vi "Main.vi"() -> ()   [LabVIEW 2012]
uses:
  States Main.ctl
  States SubVi.ctl
panel:
  out "error out":errorcluster
  in  "Exit":bool
  in  "Close":bool
  in  "Stop":bool
  in  "Open":bool
  in  "Start":bool
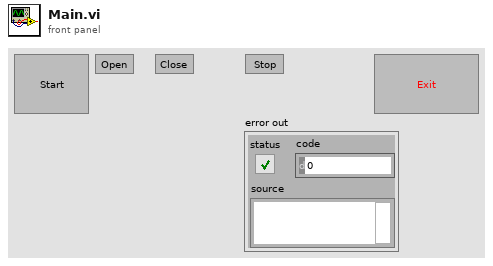
[diagram p1: front panel]
types:
  T1 = typedef "States SubVi.ctl" = enum16{"def", "Random", "Exit"}
  T2 = typedef "States Main.ctl" = enum16{"def", "Start", "Open", "Close", "Stop", "Exit"}
  T3 = enum32{"Invalid", "Standard", "Closed", "Hidden", "Minimized", "Maximized"}
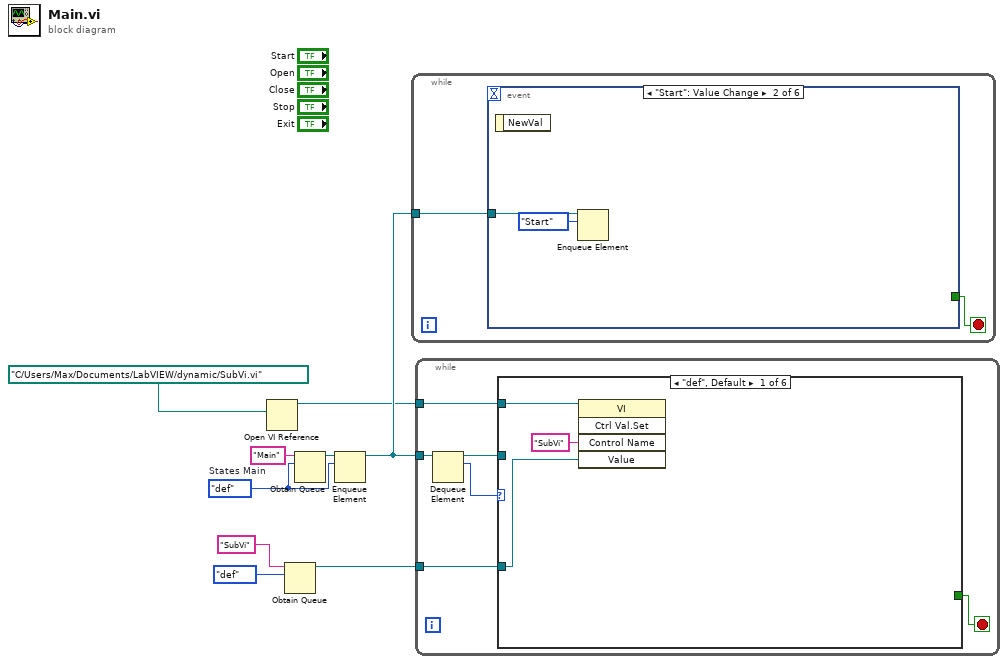
[diagram p0: block diagram]
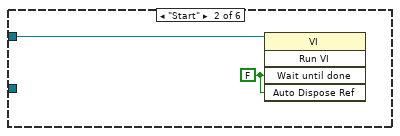
[diagram p2: hidden frame]
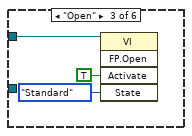
[diagram p3: hidden frame]
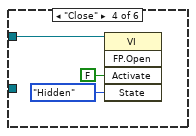
[diagram p4: hidden frame]
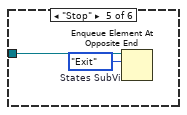
[diagram p5: hidden frame]
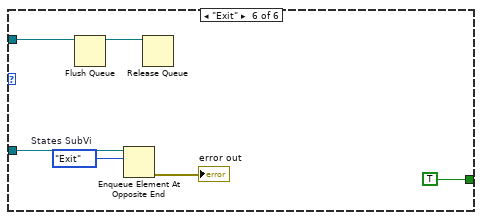
[diagram p6: hidden frame]
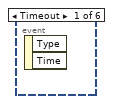
[diagram p7: hidden frame]
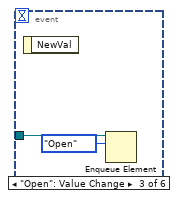
[diagram p8: hidden frame]
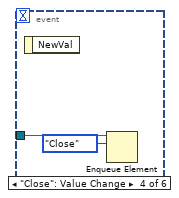
[diagram p9: hidden frame]
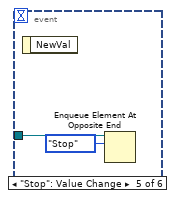
[diagram p10: hidden frame]
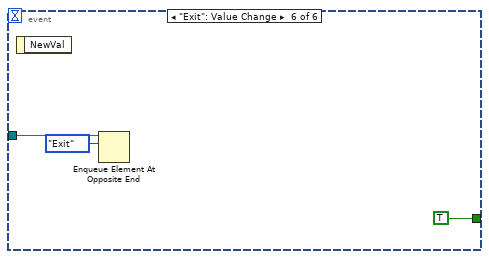
[diagram p11: hidden frame]
diagram:
  w7 = States_Main."def"  # States Main
  n1 = Open VI Reference(vi path=path "C:/Users/Max/Documents/LabVIEW/dynamic/SubVi.vi") -> (vi reference=w4:refnum<vi>)  [unwired: 5 in, 1 out]
  n2 = Obtain Queue(name (unnamed)="SubVi", element data type=States_SubVi."def" ("States SubVi")) -> (queue out=w1:refnum<queue>)  [unwired: 3 in, 2 out]
  n3 = Obtain Queue(name (unnamed)="Main", element data type=w7) -> (queue out=w8:refnum<queue>)  [unwired: 3 in, 2 out]
  n4 = Enqueue Element(queue=w8, element=w7) -> (queue out=w6:refnum<queue>)  [unwired: 2 in, 2 out]
  n5 = while {
    tunnel: w6 -> [w11]
    stop <- w10 stop-if-true
    n6 = event shown="[1] \"Start\": Value Change" {
      selector: _ -> [_ _ _ _ _ _]
      dyn-events: _ -> [_ _ _ _ _ _]
      timeout: _ -> [_ _ _ _ _ _]
      tunnel: w11 -> [_ w13 w15 w17 w19 w22]
      tunnel: [_ _ _ _ _ TRUE] -> w10
      event Timeout {
        n7 = event-data() -> ()  [unwired: 1 in, 2 out]
      }
      event "Start": Value Change {
        n8 = event-data() -> ()  [unwired: 1 in, 1 out]
        n9 = Enqueue Element(queue=w13, element=States_Main."Start") -> ()  [unwired: 2 in, 3 out]
      }
      event "Open": Value Change {
        n10 = event-data() -> ()  [unwired: 1 in, 1 out]
        n11 = Enqueue Element(queue=w15, element=States_Main."Open") -> ()  [unwired: 2 in, 3 out]
      }
      event "Close": Value Change {
        n12 = event-data() -> ()  [unwired: 1 in, 1 out]
        n13 = Enqueue Element(queue=w17, element=States_Main."Close") -> ()  [unwired: 2 in, 3 out]
      }
      event "Stop": Value Change {
        n14 = event-data() -> ()  [unwired: 1 in, 1 out]
        n15 = Enqueue Element At Opposite End(queue=w19, element=States_Main."Stop") -> ()  [unwired: 2 in, 3 out]
      }
      event "Exit": Value Change {
        n16 = event-data() -> ()  [unwired: 1 in, 1 out]
        n17 = Enqueue Element At Opposite End(queue=w22, element=States_Main."Exit") -> ()  [unwired: 2 in, 3 out]
      }
    }
  }
  n18 = while {
    tunnel: w6 -> [w28]
    tunnel: w4 -> [w26]
    tunnel: w1 -> [w23]
    stop <- w24 stop-if-true
    n19 = Dequeue Element(queue=w28) -> (queue out=w25:refnum<queue>, element=w27:T2)  [unwired: 2 in, 2 out]
    n20 = case shown="\"def\", Default" w27 {
      tunnel: w26 -> [w30 w32 w36 w39 _ _]
      tunnel: w25 -> [_ _ _ _ _ w47]
      tunnel: [_ _ _ _ _ TRUE] -> w24
      tunnel: w23 -> [w29 _ _ _ w40 w43]
      frame "def", Default {
        n21 = invoke class="VI" method="Ctrl Val.Set"(reference=w30, "Control Name"="SubVi", "Value"=w29) -> ()  [unwired: 2 in, 5 out]
      }
      frame "Start" {
        w33 = FALSE ("Wait Until Done")
        n22 = invoke class="VI" method="Run VI"(reference=w32, "Wait until done"=w33, "Auto Dispose Ref"=w33) -> ()  [unwired: 2 in, 5 out]
      }
      frame "Open" {
        n23 = invoke class="VI" method="FP.Open"(reference=w36, "Activate"=TRUE ("Activate?"), "State"=T3."Standard") -> ()  [unwired: 2 in, 5 out]
      }
      frame "Close" {
        n24 = invoke class="VI" method="FP.Open"(reference=w39, "Activate"=FALSE ("Activate?"), "State"=T3."Hidden") -> ()  [unwired: 2 in, 5 out]
      }
      frame "Stop" {
        w41 = States_SubVi."Exit"  # States SubVi
        n25 = Enqueue Element At Opposite End(queue=w40, element=w41) -> ()  [unwired: 2 in, 3 out]
      }
      frame "Exit" {
        w44 = States_SubVi."Exit"  # States SubVi
        n26 = Flush Queue(queue=w47) -> (queue out=w46:refnum<queue>)  [unwired: 1 in, 2 out]
        n27 = Enqueue Element At Opposite End(queue=w43, element=w44) -> (error out=→"error out":errorcluster)  [unwired: 2 in, 2 out]
        n28 = Release Queue(queue=w46) -> ()  [unwired: 2 in, 3 out]
      }
    }
  }
